vi "Arbiter.vi"(1 "Arbitration Type \n(Input)":T1=enum."Sum", 2 "Steps (Input)":dbl) -> (0 "Optimal Angle (Output)":dbl)   [LabVIEW 2012]
doc: "Takes in number of steps to be used, goodness functions, and arbitration type. Sends angles to gfunctions, takes weighted (based on arbitration type) sum and outputs angle from northing that is optimal."
uses:
  ArbitrationType.ctl
panel:
  out "Array":dbl[](array[numeric])
  out "appended array":dbl[][](array[numeric])
  # "Arbiter: Takes in Steps, Arbitration Type, Outputs Optimal Angle"
  # "Degrees from Northing, Clockwise"
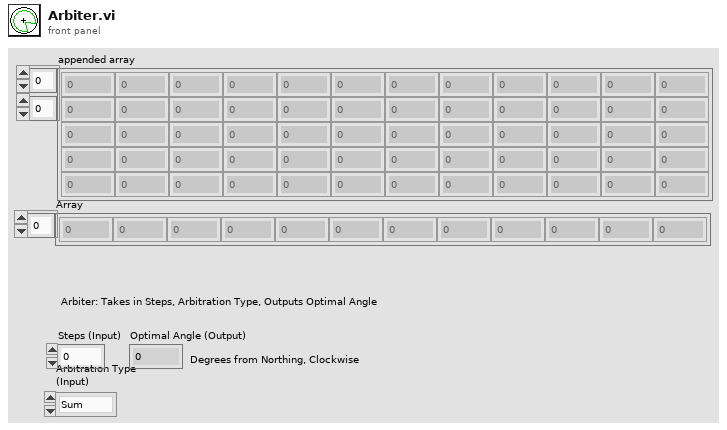
[diagram p1: front panel]
types:
  T1 = typedef "ArbitrationType.ctl" = enum16{"Product", "Sum", "Maximum"}
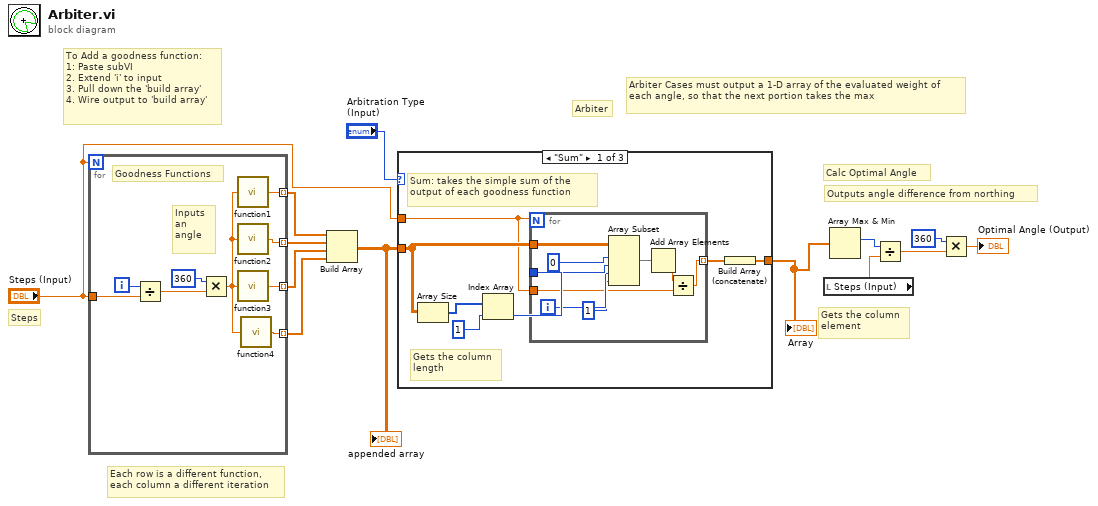
[diagram p0: block diagram]
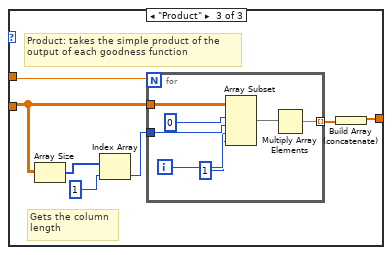
[diagram p3: hidden frame]
diagram:
  # "Outputs angle difference from northing"
  # "Calc Optimal Angle"
  # "Gets the column\nelement"
  # "Arbiter Cases must output a 1-D array of the evaluated weight of each angle, so that the next portion takes the max"
  # "Arbiter"
  # "To Add a goodness function:\n1: Paste subVI\n2. Extend 'i' to input\n3. Pull down the 'build array'\n4. Wire output to 'build array'"
  # "Each row is a different function,\neach column a different iteration"
  # "Steps"
  n1 = for {
    N: "Steps (Input)" -> [_]
    tunnel: [w22] -> w11 mode=indexing
    tunnel: [w21] -> w12 mode=indexing
    tunnel: [w20] -> w13 mode=indexing
    tunnel: "Steps (Input)" -> [w18]
    tunnel: [w14] -> w2 mode=indexing
    i -> [w19]
    # "Goodness Functions"
    # "Inputs an angle"
    n2 = Divide(x=w19, y=w18) -> (x/y=w17:dbl)
    n3 = Multiply(x=360, y=w17) -> (x*y=w15:dbl)
    n4 = call "function1.vi"("y"=w15) -> ("x+y"=w22:dbl)
    n5 = call "function2.vi"("y"=w15) -> ("x+y"=w21:dbl)
    n6 = call "function3.vi"("y"=w15) -> ("x+y"=w20:dbl)
    n7 = call "function4.vi"("Input"=w15) -> ("Output"=w14:dbl)
  }
  n8 = Build Array(w11, w12, w13, w2) -> (w5:dbl[][])
  "appended array" <- w5
  n9 = case shown="\"Sum\"" "Arbitration Type \n(Input)" {
    tunnel: w5 -> [w29 _ w41]
    tunnel: [w28 _ w40] -> w4
    tunnel: "Steps (Input)" -> [w23 _ w42]
    frame "Sum" {
      # "Sum: takes the simple sum of the output of each goodness function"
      # "Gets the column\nlength"
      n10 = Array Size(array=w29) -> (size(s)=w27:i32[])
      n11 = Index Array(array=w27, index=1) -> (element=w25:i32)
      n12 = for {
        N: w23 -> [_]
        tunnel: w29 -> [w38]
        tunnel: [w31] -> w24 mode=indexing
        tunnel: w25 -> [w35]
        tunnel: w23 -> [w30]
        i -> [w34]
        n13 = Array Subset(array=w38, index (row)=0, length (row)=w35, index (col)=w34, length (col)=1) -> (w37:dbl[][])
        n14 = Add Array Elements(numeric array=w37) -> (sum=w32:dbl)
        n15 = Divide(x=w32, y=w30) -> (x/y=w31:dbl)
      }
      n16 = Build Array (concatenate)(w24) -> (w28:dbl[])
    }
    frame "Maximum" {
    }
    frame "Product" {
      # "Product: takes the simple product of the output of each goodness function"
      # "Gets the column\nlength"
      n17 = Array Size(array=w41) -> (size(s)=w45:i32[])
      n18 = Index Array(array=w45, index=1) -> (element=w43:i32)
      n19 = for {
        N: w42 -> [_]
        tunnel: w41 -> [w52]
        tunnel: w43 -> [w50]
        tunnel: [w46] -> w39 mode=indexing
        i -> [w49]
        n20 = Array Subset(array=w52, index (row)=0, length (row)=w50, index (col)=w49, length (col)=1) -> (w47:dbl[][])
        n21 = Multiply Array Elements(1:w47) -> (0:w46:dbl)
      }
      n22 = Build Array (concatenate)(w39) -> (w40:dbl[])
    }
  }
  "Array" <- w4
  n23 = local read "Steps (Input)"() -> (w6:dbl)
  n24 = Array Max & Min(array=w4) -> (max index (indices)=w3:i32)  [unwired: 3 out]
  n25 = Divide(x=w3, y=w6) -> (x/y=w7:dbl)
  n26 = Multiply(x=360, y=w7) -> (x*y=→"Optimal Angle (Output)":dbl)
